vi "Calc.vi"   [LabVIEW 2018]
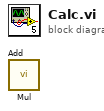
[diagram p0: block diagram]
diagram:
  n1 = call "Mul.vi"() -> ()  [unwired: 11 in, 1 out]
  n2 = call "Add.vi"() -> ()  [unwired: 11 in, 1 out]
